vi "setStep.vi"(8 "error in (no error)":errorcluster, 9 "Step Value":dbl, 10 "Axis Letter":string, 11 "Controller in":refnum<class "Controller.lvclass">) -> (0 "error out":errorcluster, 3 "Controller out":refnum<class "Controller.lvclass">)   [LabVIEW 2019, in "Controller.lvclass"]
uses:
  Controller.lvclass
  Axis/Axis.lvclass
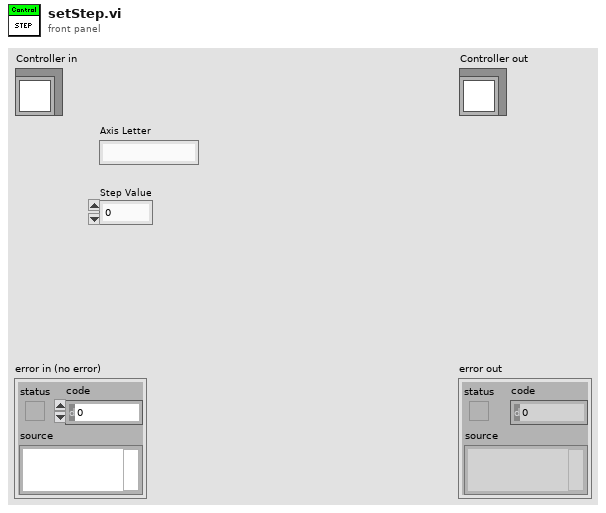
[diagram p1: front panel]
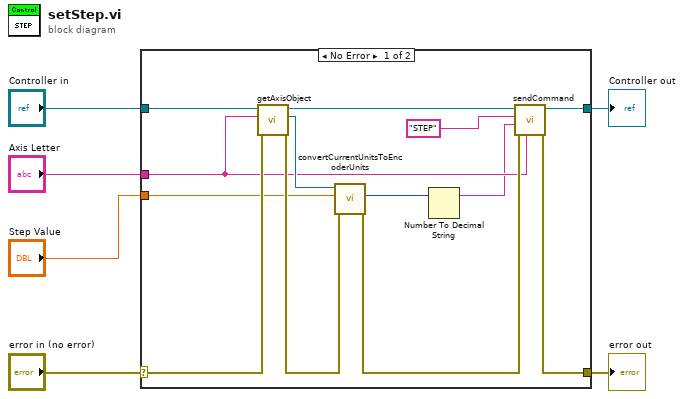
[diagram p0: block diagram]
diagram:
  n1 = case shown="No Error" "error in (no error)" {
    selector: "error in (no error)" -> [w11 w21]
    tunnel: [w13 w21] -> w5
    tunnel: [w14 w20] -> w3
    tunnel: "Controller in" -> [w19 w20]
    tunnel: "Axis Letter" -> [w8 _]
    tunnel: "Step Value" -> [w10 _]
    frame No Error {
      n2 = call-dynamic "getAxisObject.vi"("error in (no error)"=w11, "Axis Letter"=w8, "Controller in"=w19) -> ("error out"=w17:errorcluster, "Axis Object"=w18:refnum<class "Axis.lvclass">, "Controller out"=w15:refnum<class "Controller.lvclass">)  [unwired: 6 in]
      n3 = call-dynamic "convertCurrentUnitsToEncoderUnits.vi"("error in (no error)"=w17, "Value In Current Units"=w10, "Axis in"=w18) -> ("error out"=w16:errorcluster, "Value In Encoder Units"=w9:i32)  [unwired: 6 in, 1 out]
      n4 = Number To Decimal String(number=w9) -> (decimal integer string=w7:string)  [unwired: 1 in]
      n5 = call-dynamic "sendCommand.vi"("Axis Letter"=w8, "error in (no error)"=w16, "Value"=w7, "Command"="STEP", "Controller in"=w15) -> ("error out"=w13:errorcluster, "Controller out"=w14:refnum<class "Controller.lvclass">)  [unwired: 5 in]
    }
    frame Error {
    }
  }
  "error out" <- w5
  "Controller out" <- w3
